vi "Smart Open.vi"(7 "Allow multiple opens?":bool=TRUE, 8 "error in (no error)":errorcluster, 10 "Channel Name":tag) -> (0 "error out":errorcluster, 3 "SPI Ref Out":T1={"myRIO Reference"={"myRIO Model"=enum."Unknown", "myRIO Hardware Reference"={"Generic FPGA Reference"=refnum, "Allow multiple opens"=FALSE}}, "SPI Channels Enum"=enum."Not Connected", "SPI Configuration"={"Frequency [Hz]"=0.0, "Clock Phase"=enum."Leading", "Clock Polarity"=enum."Low", "Data Direction"=enum."Most significant bit first", "Frame Length"=8}} {"SPI Configuration"."Frame Length" min=1 max=16})   [LabVIEW 2021, in "SPI.lvlib"]
uses:
  <vilib>/myRIO/Instrument Drivers/Onboard IO/SPI/SPI.lvlib
  <vilib>/myRIO/Common/Instrument Driver Framework/Utilities/typedefs/Hardware Version Enum.ctl
  <vilib>/myRIO/Common/Instrument Driver Framework/Utilities/typedefs/Generic FPGA Reference.ctl
  <vilib>/myRIO/Common/Instrument Driver Framework/myRIO v1.0/SPI/typedefs/SPI Channels Enum.ctl
  <vilib>/myRIO/Common/Instrument Driver Framework/myRIO v1.0/SPI/typedefs/SPI Clock Phase.ctl
  <vilib>/myRIO/Common/Instrument Driver Framework/myRIO v1.0/SPI/typedefs/SPI Clock Polarity.ctl
  <vilib>/myRIO/Common/Instrument Driver Framework/myRIO v1.0/SPI/typedefs/SPI Data Direction.ctl
  <vilib>/myRIO/Common/Instrument Driver Framework/myRIO v1.0/SPI/typedefs/SPI Frame Length.ctl
  <vilib>/myRIO/Instrument Drivers/Onboard IO/SPI/typedefs/SPI Reference.ctl
  <vilib>/myRIO/Common/Instrument Driver Framework/Utilities/typedefs/myRIO v1.0 Reference.ctl
  <vilib>/myRIO/Common/Instrument Driver Framework/Utilities/typedefs/myRIO Generic Hardware Reference.ctl
  <vilib>/myRIO/Instrument Drivers/Onboard IO/SPI/typedefs/SPI Configuration.ctl
  <vilib>/myRIO/Instrument Drivers/Onboard IO/SPI/vis/myRIO SPI Open.xnode
  <vilib>/myRIO/Common/Instrument Driver Framework/myRIO v1.0/SPI/vis/myRIO v1.1 Open SPI.vi
  <vilib>/userdefined/High Color/nirio_resource_hc.ctl
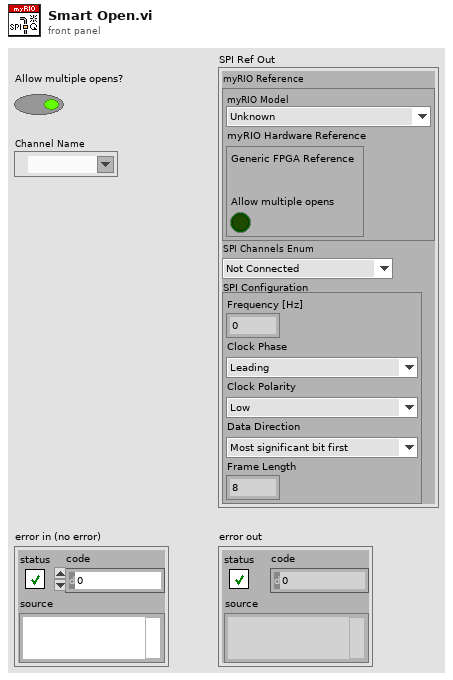
[diagram p1: front panel]
types:
  T1 = typedef "SPI.lvlib/SPI Reference.ctl" = cluster{"myRIO Reference":T2, "SPI Channels Enum":T6, "SPI Configuration":T7}
  T2 = typedef "myRIO Generic Hardware Reference.ctl" = cluster{"myRIO Model":T3, "myRIO Hardware Reference":T4}
  T3 = typedef "Hardware Version Enum.ctl" = enum16{"Unknown", "myRIO-1900", "myRIO-1950", "roboRIO", "NI ELVIS RIO CM", "ELVIS III"}
  T4 = typedef "myRIO v1.0 Reference.ctl" = cluster{"Generic FPGA Reference":T5, "Allow multiple opens":bool}
  T5 = typedef "Generic FPGA Reference.ctl" = refnum<k20>
  T6 = typedef "SPI Channels Enum.ctl" = enum16{"Not Connected", "A/SPI", "B/SPI", "SPI/SPI"}
  T7 = typedef "SPI.lvlib/SPI Configuration.ctl" = cluster{"Frequency [Hz]":dbl, "Clock Phase":T8, "Clock Polarity":T9, "Data Direction":T10, "Frame Length":T11}
  T8 = typedef "SPI Clock Phase.ctl" = enum8{"Leading", "Trailing"}
  T9 = typedef "SPI Clock Polarity.ctl" = enum8{"Low", "High"}
  T10 = typedef "SPI Data Direction.ctl" = enum8{"Most significant bit first", "Least significant bit first"}
  T11 = typedef "SPI Frame Length.ctl" = u8
  T12 = typedef "nirio_resource_hc.ctl" = tag
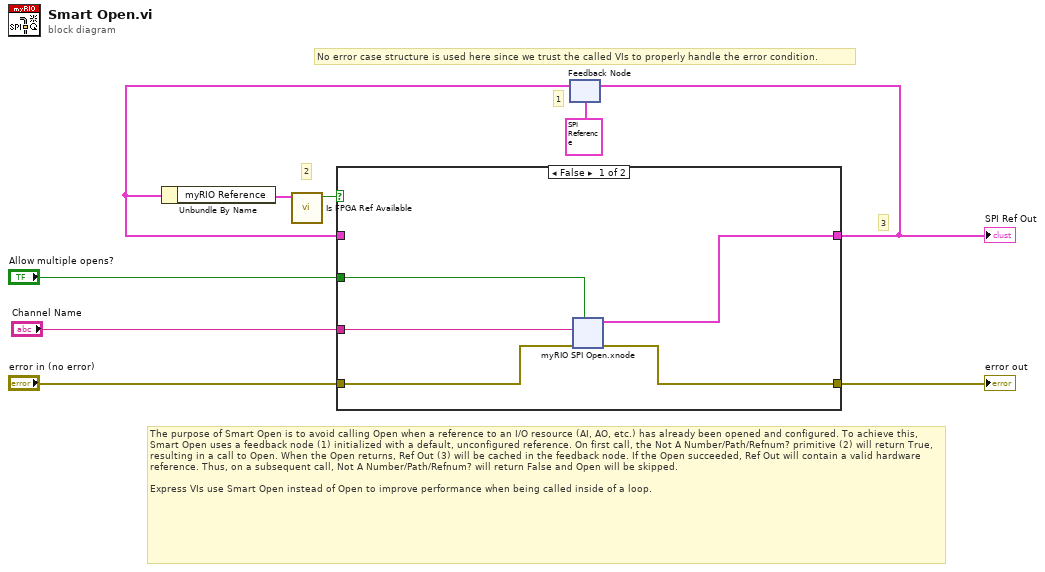
[diagram p0: block diagram]
diagram:
  # "No error case structure is used here since we trust the called VIs to properly handle the error condition."
  # "2"
  # "1"
  # "3"
  # "The purpose of Smart Open is to avoid calling Open when a reference to an I/O resource (AI, AO, etc.) has already been opened and configured. To achieve this, Smart Open uses a feedback node (1) initialized with a default, unconfigured reference. On first call, the Not A Number/Path/Refnum? primitive (2) will return True, resulting in a call to Open. When the Open returns, Ref Out (3) will be cached in the feedback node. If the Open succeeded, Ref Out will contain a valid hardware reference. Thus, on a subsequent call, Not A Number/Path/Refnum? will return False and Open will be skipped.\n\t\nExpress VIs use Smart Open instead of Open to improve performance when being called inside of a loop."
  n1 = feedback #1(T1 {"myRIO Reference"={"myRIO Model"=enum."Unknown", "myRIO Hardware Reference"={"Generic FPGA Reference"=refnum, "Allow multiple opens"=FALSE}}, "SPI Channels Enum"=enum."Not Connected", "SPI Configuration"={"Frequency [Hz]"=0.0, "Clock Phase"=enum."Leading", "Clock Polarity"=enum."Low", "Data Direction"=enum."Most significant bit first", "Frame Length"=0}} ("AI Ref Out")) -> (w4:T1)
  n2 = Unbundle By Name(w4) -> ("myRIO Reference"=w1:T2)
  n3 = call <vilib>:"Is FPGA Ref Available.vi"("myRIO Reference"=w1) -> ("Is Available?"=w5:bool)  [unwired: 10 in]
  n4 = case shown="False" w5 {
    tunnel: "error in (no error)" -> [w14 w31]
    tunnel: [w13 w32] -> w7
    tunnel: [w12 w31] -> w8
    tunnel: w4 -> [_ w32]
    tunnel: "Allow multiple opens?" -> [w11 _]
    tunnel: "Channel Name" -> [w10 _]
    frame False {
      n5 = xnode "myRIO SPI Open.xnode"("error in (no error)"=w14, "Allow multiple opens?"=w11, "Channel Name"=w10) -> ("error out"=w12:errorcluster, "SPI Ref Out"=w13:T1)
    }
    frame True {
    }
  }
  "SPI Ref Out" <- w7
  "error out" <- w8
  n6 = feedback-in #1(w7) -> ()
